vi "GetSpecificControl.vi"(8 "error in (no error)":errorcluster, 10 "Name":string, 11 "VIEW in":refnum<class "VIEW.lvclass">) -> (0 "error out":errorcluster, 2 "output cluster":T1, 3 "VIEW out":refnum<class "VIEW.lvclass">)   [LabVIEW 2013, in "VIEW.lvclass"]
uses:
  VIEW.lvclass
  VIEW.lvclass/VIEW.ctl
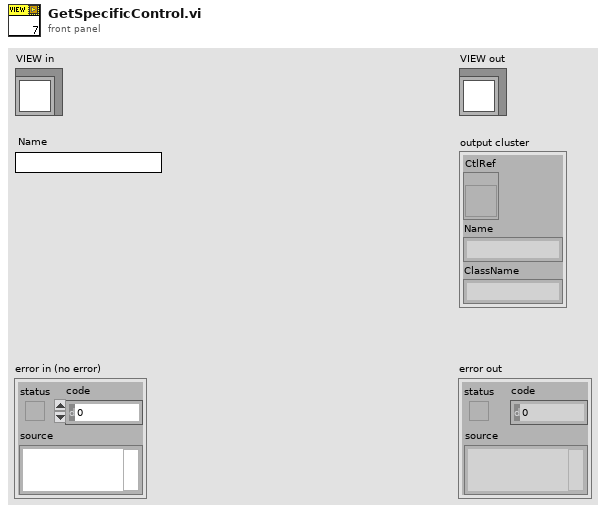
[diagram p1: front panel]
types:
  T1 = cluster{"CtlRef":refnum<vi>, "Name":string, "ClassName":string}
  T2 = cluster{"CtlRef":refnum<vi>, "Name":string, "ClassName":string}[]
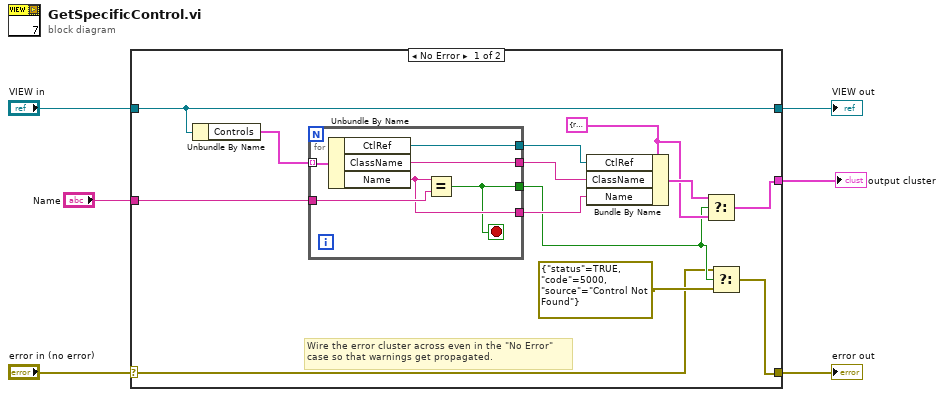
[diagram p0: block diagram]
diagram:
  n1 = case shown="No Error" "error in (no error)" {
    selector: "error in (no error)" -> [w8 w27]
    tunnel: [w7 w27] -> w5
    tunnel: [w19 w26] -> w3
    tunnel: "VIEW in" -> [w19 w26]
    tunnel: "Name" -> [w17 _]
    tunnel: [w11 _] -> w1
    frame No Error {
      w12 = T1 {"CtlRef"=refnum, "Name"="", "ClassName"=""} ("CtlInfo")
      # "Wire the error cluster across even in the \"No Error\"\ncase so that warnings get propagated."
      n2 = Unbundle By Name(w19) -> ("Controls"=w18:T2)
      n3 = for {
        tunnel: w18 -> [w25] mode=indexing
        tunnel: w17 -> [w24]
        tunnel: [w23] -> w16
        tunnel: [w22] -> w15
        tunnel: [w21] -> w14
        tunnel: [w20] -> w10
        stop <- w20 stop-if-true
        n4 = Unbundle By Name(w25) -> ("CtlRef"=w23:refnum<vi>, "ClassName"=w22:string, "Name"=w21:string)
        n5 = Equal?(x=w21, y=w24) -> (x = y?=w20:bool)
      }
      n6 = Bundle By Name(cluster=w12, "CtlRef"=w16, "ClassName"=w15, "Name"=w14) -> (w13:T1)
      n7 = Select(t=w13, s=w10, f=w12) -> (s? t:f=w11:T1)
      n8 = Select(t=w8, s=w10, f=errorcluster {"status"=TRUE, "code"=5000, "source"="Control Not Found"}) -> (s? t:f=w7:errorcluster)
    }
    frame Error {
    }
  }
  "error out" <- w5
  "VIEW out" <- w3
  "output cluster" <- w1
